vi "Read Digital Voltmeter MDO3034.vi"(8 "error in (no error)":errorcluster, 11 "VISA resource name":refnum<visa-resource-name>) -> (0 "error out":errorcluster, 2 "Digital Voltmeter Value":dbl, 3 "VISA resource name out":refnum<visa-resource-name>)   [LabVIEW 2021]
doc: "Reads the current value and frequency for the Digital Voltmeter.\n\n<B>Notes:</B>\n(1) This VI is available for MDO3000 and MDO3 Series only.\n\n(2) Requires the MDO3DVM option to be installed for MDO3000 and 3-DVM option to be installed for MDO3."
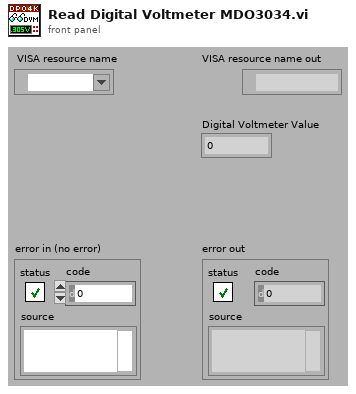
[diagram p1: front panel]
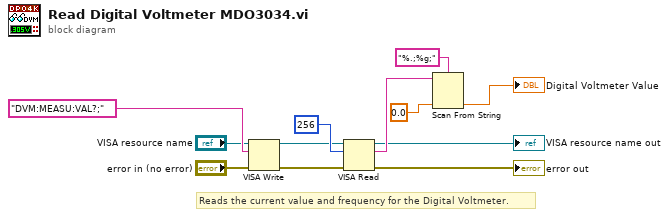
[diagram p0: block diagram]
diagram:
  # "Reads the current value and frequency for the Digital Voltmeter."
  n1 = VISA Write(VISA resource name="VISA resource name", write buffer="DVM:MEASU:VAL?;", error in (no error)="error in (no error)") -> (VISA resource name out=w2:refnum<visa-resource-name>, error out=w1:errorcluster)  [unwired: 1 out]
  n2 = VISA Read(VISA resource name=w2, byte count=u32 256, error in (no error)=w1) -> (VISA resource name out=→"VISA resource name out":refnum<visa-resource-name>, read buffer=w8:string, error out=→"error out":errorcluster)  [unwired: 1 out]
  n3 = Scan From String(format string="%.;%g;", input string=w8, default 1=0.0 ("default value 1")) -> (output 1=→"Digital Voltmeter Value":dbl)  [unwired: 2 in, 3 out]
